vi "Eliminated.vi"(6 "Column":i32, 8 "Row":i32, 9 "Killer":i32, 10 "Team":i32, 11 "SquareA in":refnum<class "Ant Mound.lvclass">) -> (3 "SquareA out":refnum<class "Ant Mound.lvclass">)   [LabVIEW 2015, in "Ant Mound.lvclass"]
uses:
  Ant Mound.lvclass
  Square/Square.lvclass
  Common/Location Data.ctl
  Common/Common.lvlib
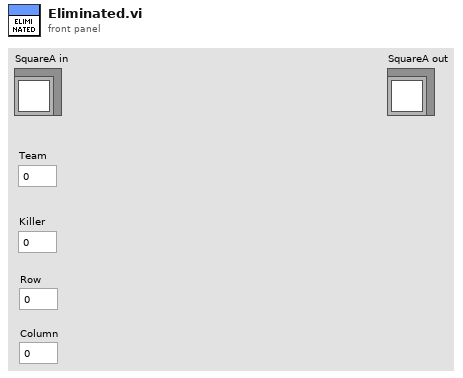
[diagram p1: front panel]
types:
  T1 = typedef "Common.lvlib/Map DVR.ctl" = refnum<data-value>
  T2 = typedef "Common.lvlib/Location Data.ctl" = cluster{"Location State":enum16{"Empty", "Enemy", "Attacked", "Occupied"}, "Round Updated":i32}
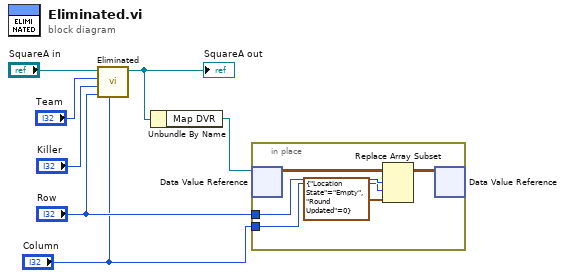
[diagram p0: block diagram]
diagram:
  n1 = call-parent "Eliminated.vi"("Column"="Column", "Row"="Row", "Killer"="Killer", "Team"="Team", "Square in"="SquareA in") -> ("Square out"=w4:refnum<class "Ant Mound.lvclass">)  [unwired: 6 in]
  "SquareA out" <- w4
  n2 = Unbundle By Name(w4) -> ("Map DVR"=w3:T1)
  n3 = in-place {
    in-place-border: "Row" -> [w10]
    in-place-border: "Column" -> [w9]
    n4 = in-place-dvr #1(w3) -> (w12:T2[][])  [unwired: 1 out]
    n5 = Replace Array Subset(array=w12, new element=T2 {"Location State"=enum."Empty", "Round Updated"=0} ("new element/subarray"), index (row)=w10, index (col)=w9) -> (w11:T2[][])
    n6 = in-place-dvr #1(w11) -> ()  [unwired: 2 out]
  }
